vi "RanLate_.vi"() -> ()   [LabVIEW 2017]
uses:
  <vilib>/Platform/TimedLoop/XDataNode/timing_clust.ctl
  <vilib>/Platform/TimedLoop/XDataNode/nitl_modes.ctl
  <vilib>/Platform/TimedLoop/XDataNode/wakeup.ctl
  <vilib>/platform/TimedLoop/XDataNode/XDataNode.xnode
  <vilib>/Platform/TimedLoop/XDataNode/XDNodeRunTimeDep.lvlib
  <resource>/objmgr/nimcai.rc
panel:
  out "Execution times (us)":dbl[](graph)
  out "max value":dbl
  out "Position Feedback":dbl
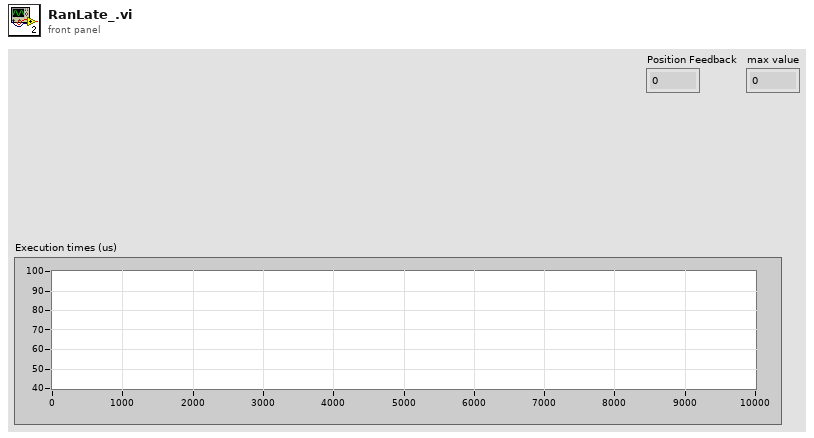
[diagram p1: front panel]
types:
  T1 = typedef "XDNodeRunTimeDep.lvlib/timing_clust.ctl" = cluster{"Expected End [f-1]":u64, "Actual End [f-1]":u64, "Finished Late? [f-1]":bool, "Expected End [i-1]":u64, "Actual End [i-1]":u64, "Finished Late? [i-1]":bool, "Expected Start [i]":u64, "Actual Start [i]":u64, "Expected Start [f]":u64, "Actual Start [f]":u64, "Source Name":string, "Structure Name":string, "Period":i64, "Deadline":i64, "Offset":i64, "Start":i64, "Priority":i32, "Timeout":i32, "Mode":T2, "Wakeup Reason":T3, "Error":errorcluster, "Source Type":string, "Secondary Source Type":string, "Global End Time":u64, "Global Start Time":u64, "Frame Duration":u64, "Iteration Duration":u64, "Assigned CPU":i32, "I/O Scan Engine Mode":u32}
  T2 = typedef "XDNodeRunTimeDep.lvlib/nitl_modes.ctl" = enum32{"No Change", "Process missed periods, maintain original phase", "Discard missed periods, maintain original phase", "Process missed periods, ignore original phase", "Discard missed periods, ignore original phase"}
  T3 = typedef "XDNodeRunTimeDep.lvlib/wakeup.ctl" = enum32{"Normal", "Aborted", "Asynchronous wakeup", "Timing source error", "Timed loop error", "Timeout"}
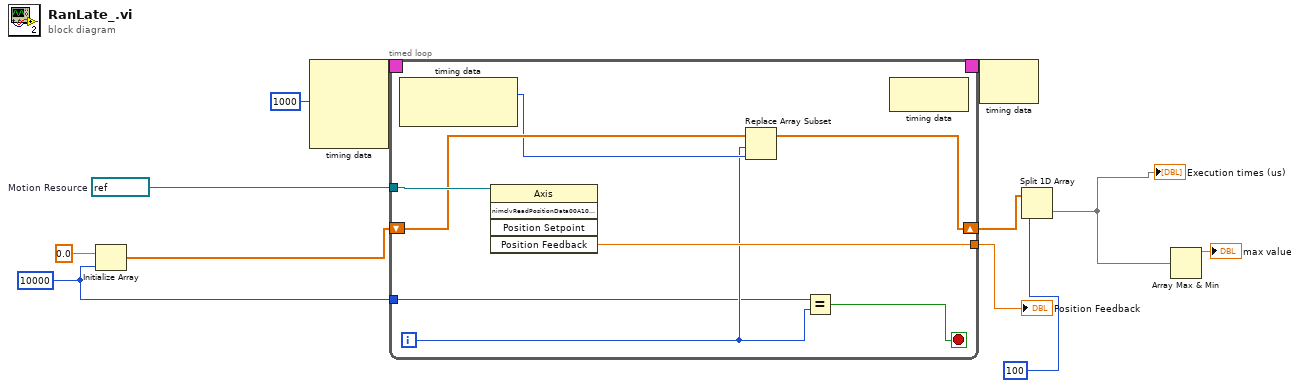
[diagram p0: block diagram]
diagram:
  w5 = 10000 ("dimension size")
  w10 = refnum<k21> "Axis 1"  # Motion Resource
  n1 = Initialize Array(0.0 ("element"), w5) -> (w6:dbl[])
  n2 = node-c288(i64 1000 ("Period")) -> (w12:T1)  [unwired: 3 in]
  n3 = timed-loop {
    timing: w12 -> [_]
    timing-out: [_] -> w11
    tunnel: w10 -> [w20]
    tunnel: [w19] -> w9
    shift-right: [w16] -> w3
    shift-left: w6 -> [w18]
    tunnel: w5 -> [w14]
    i -> [w15]
    stop <- w13 stop-if-true
    n4 = node-c288() -> (w17:i64)  [unwired: 1 in, 1 out]
    n5 = invoke class="Axis" method="nimclvReadPositionData00A10001"(reference=w20) -> ("Position Feedback"=w19:dbl)  [unwired: 4 in, 4 out]
    n6 = Replace Array Subset(array=w18, new element=w17, index=w15) -> (w16:dbl[])
    n7 = Equal?(x=w14, y=w15) -> (x = y?=w13:bool)
    n8 = node-c288() -> ()  [unwired: 1 in, 1 out]
  }
  "Position Feedback" <- w9
  n9 = node-c288(w11) -> ()  [unwired: 1 out]
  n10 = Split 1D Array(array=w3, index=100) -> (second subarray=w1:dbl[])  [unwired: 1 out]
  "Execution times (us)" <- w1
  n11 = Array Max & Min(array=w1) -> (max value=→"max value":dbl)  [unwired: 3 out]
